vi "Global.vi"() -> ()   [LabVIEW 2019]
panel:
  in  "Joystick X":dbl
  in  "AngleStartTurn":dbl
  in  "RobotStartAngle":dbl
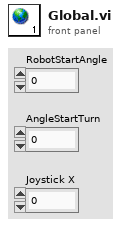
[diagram p1: front panel]
diagram:
